vi "Sub_predictor_v3(SubVI).vi"(6 "predicted step":dbl=0.04 format="%#_13g", 8 "Sim_running":bool, 9 "q_i":dbl[](array[numeric]), 11 "t [s]":dbl) -> (0 "Euler Angles Table [deg]":dbl[](array[numeric]), 3 "Euler Angles Table_pred [deg]":dbl[](array[numeric]))   [LabVIEW 2017]
uses:
  <vilib>/Analysis/coordinate.llb/Euler Rotation Order.ctl
  <vilib>/Analysis/7linalg.llb/Real Transpose Matrix.vi
  <vilib>/Analysis/_algsub.llb/Real PseudoInverse Matrix.vi
  <vilib>/Analysis/baseanly.llb/Real A x B.vi
  <vilib>/Analysis/Matrix/Numeric/Conversions/Array To Matrix - RA2.vi
  <vilib>/Analysis/Matrix/Numeric/Conversions/Array To Matrix - RA.vi
  <vilib>/Analysis/Matrix/Numeric/Conversions/Matrix To Array - RM.vi
  <vilib>/Analysis/Matrix/NI_Matrix.lvlib
  <vilib>/Analysis/NI_AALPro.lvlib
  <vilib>/Analysis/NI_AALBase.lvlib
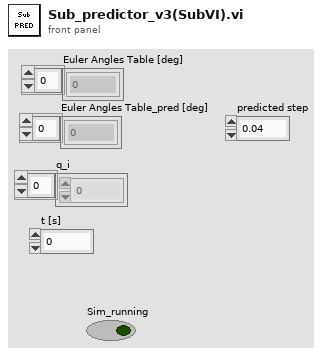
[diagram p1: front panel]
types:
  T1 = typedef "NI_AALPro.lvlib/Euler Rotation Order.ctl" = u16
  T2 = typedef "NI_Matrix.lvlib/RealMatrix.ctl" = dbl[][]
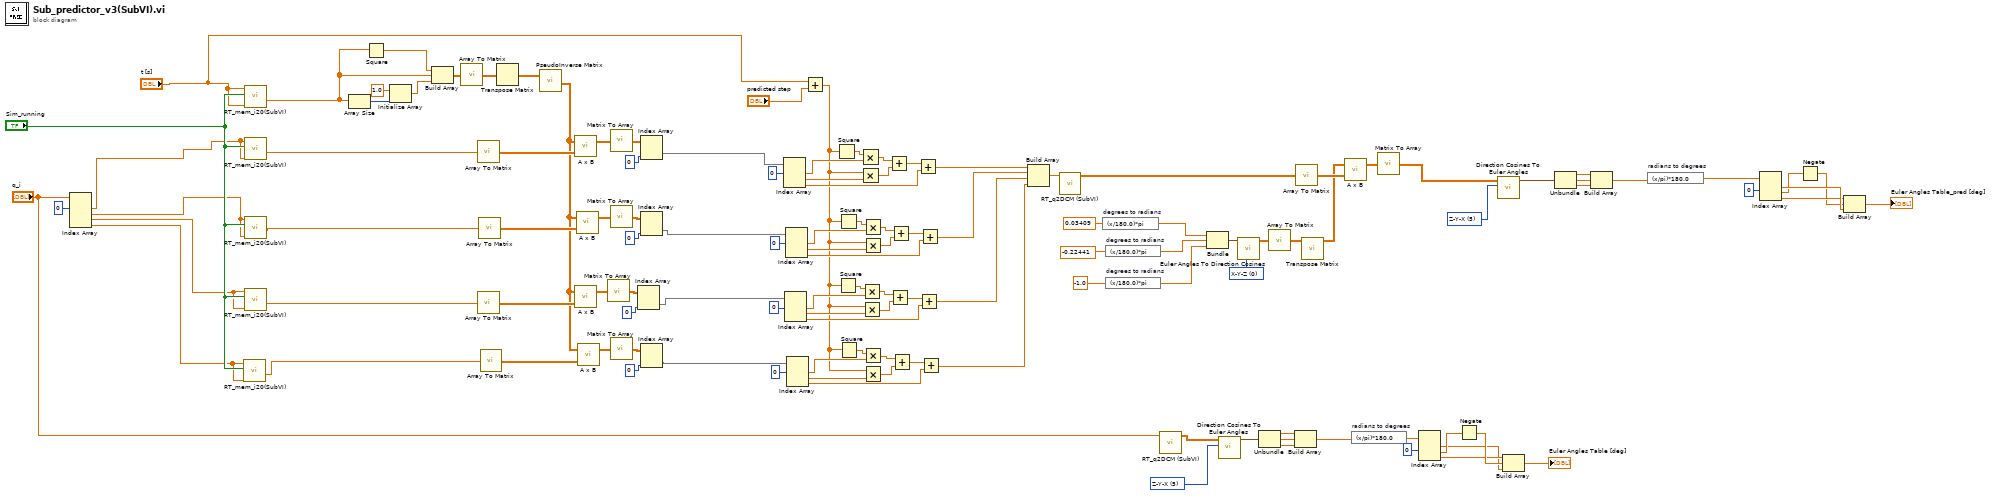
[diagram p0: block diagram]
diagram:
  w14 = T1 0 items=["X-Y-Z", "X-Z-Y", "Y-X-Z", "Y-Z-X", "Z-X-Y", "Z-Y-X", "X-Y-X", "X-Z-X", "Y-X-Y", "Y-Z-Y", "Z-X-Z", "Z-Y-Z"] ("rotation order")
  w17 = T1 5 items=["X-Y-Z", "X-Z-Y", "Y-X-Z", "Y-Z-X", "Z-X-Y", "Z-Y-X", "X-Y-X", "X-Z-X", "Y-X-Y", "Y-Z-Y", "Z-X-Z", "Z-Y-Z"] ("rotation order")
  w43 = T1 5 items=["X-Y-Z", "X-Z-Y", "Y-X-Z", "Y-Z-X", "Z-X-Y", "Z-Y-X", "X-Y-X", "X-Z-X", "Y-X-Y", "Y-Z-Y", "Z-X-Z", "Z-Y-Z"] ("rotation order")
  n1 = Index Array(array="q_i", index #1=0 ("index")) -> (element #1=w92:dbl, element #2=w91:dbl, element #3=w90:dbl, element #4=w89:dbl)  [unwired: 3 in]
  n2 = call "RT_mem_i20(SubVI).vi"("Ini_val"=w89, "start"="Sim_running", "In"=w89) -> ("in_vec"=w95:dbl[])  [unwired: 7 in, 1 out]
  n3 = call "RT_mem_i20(SubVI).vi"("Ini_val"="t [s]", "start"="Sim_running", "In"="t [s]") -> ("in_vec"=w103:dbl[])  [unwired: 7 in, 1 out]
  n4 = call "RT_mem_i20(SubVI).vi"("Ini_val"=w92, "start"="Sim_running", "In"=w92) -> ("in_vec"=w115:dbl[])  [unwired: 7 in, 1 out]
  n5 = call "RT_mem_i20(SubVI).vi"("Ini_val"=w91, "start"="Sim_running", "In"=w91) -> ("in_vec"=w112:dbl[])  [unwired: 7 in, 1 out]
  n6 = call "RT_mem_i20(SubVI).vi"("Ini_val"=w90, "start"="Sim_running", "In"=w90) -> ("in_vec"=w116:dbl[])  [unwired: 7 in, 1 out]
  n7 = Array Size(array=w103) -> (size(s)=w100:i32)
  n8 = Square(x=w103) -> (x^2=w102:dbl[])
  n9 = Initialize Array(1.0 ("element"), w100) -> (w104:dbl[])
  n10 = Build Array(w102, w103, w104) -> (w106:dbl[][])
  n11 = call-poly <vilib>:"Array To Matrix.vi"("Real 2D Array"=w106) -> ("Real Matrix"=w105:T2)
  n12 = call-poly <vilib>:"Array To Matrix.vi"("Real 1D Array"=w115) -> ("Real Matrix (Column Vector)"=w113:T2)
  n13 = call-poly <vilib>:"Array To Matrix.vi"("Real 1D Array"=w116) -> ("Real Matrix (Column Vector)"=w114:T2)
  n14 = call-poly <vilib>:"Array To Matrix.vi"("Real 1D Array"=w112) -> ("Real Matrix (Column Vector)"=w108:T2)
  n15 = call-poly <vilib>:"Array To Matrix.vi"("Real 1D Array"=w95) -> ("Real Matrix (Column Vector)"=w99:T2)
  n16 = Transpose Matrix(1:w105) -> (0:w107:T2)
  n17 = call-poly <vilib>:"PseudoInverse Matrix.vi"("Input Matrix"=w107) -> ("PseudoInverse Matrix"=w94:T2)  [unwired: 1 in, 1 out]
  n18 = call-poly <vilib>:"A x B.vi"("B"=w113, "A"=w94) -> ("A x B"=w121:T2)  [unwired: 1 out]
  n19 = call-poly <vilib>:"A x B.vi"("B"=w114, "A"=w94) -> ("A x B"=w122:T2)  [unwired: 1 out]
  n20 = call-poly <vilib>:"A x B.vi"("B"=w108, "A"=w94) -> ("A x B"=w111:T2)  [unwired: 1 out]
  n21 = call-poly <vilib>:"A x B.vi"("B"=w99, "A"=w94) -> ("A x B"=w96:T2)  [unwired: 1 out]
  n22 = call-poly <vilib>:"Matrix To Array.vi"("Real Matrix"=w122) -> ("Real 2D Array"=w119:dbl[][])
  n23 = call-poly <vilib>:"Matrix To Array.vi"("Real Matrix"=w121) -> ("Real 2D Array"=w118:dbl[][])
  n24 = call-poly <vilib>:"Matrix To Array.vi"("Real Matrix"=w111) -> ("Real 2D Array"=w109:dbl[][])
  n25 = call-poly <vilib>:"Matrix To Array.vi"("Real Matrix"=w96) -> ("Real 2D Array"=w98:dbl[][])
  n26 = Index Array(array=w119, index (col)=0 ("index (row)")) -> (element=w51:dbl[])  [unwired: 1 in]
  n27 = Index Array(array=w118, index (col)=0 ("index (row)")) -> (element=w78:dbl[])  [unwired: 1 in]
  n28 = Index Array(array=w109, index (col)=0 ("index (row)")) -> (element=w52:dbl[])  [unwired: 1 in]
  n29 = Index Array(array=w98, index (col)=0 ("index (row)")) -> (element=w50:dbl[])  [unwired: 1 in]
  n30 = Index Array(array=w78, index #1=0 ("index")) -> (element #1=w81:dbl, element #2=w83:dbl, element #3=w86:dbl)  [unwired: 2 in]
  n31 = Index Array(array=w51, index #1=0 ("index")) -> (element #1=w63:dbl, element #2=w65:dbl, element #3=w68:dbl)  [unwired: 2 in]
  n32 = Index Array(array=w52, index #1=0 ("index")) -> (element #1=w74:dbl, element #2=w72:dbl, element #3=w69:dbl)  [unwired: 2 in]
  n33 = Index Array(array=w50, index #1=0 ("index")) -> (element #1=w58:dbl, element #2=w56:dbl, element #3=w53:dbl)  [unwired: 2 in]
  n34 = Add(x="t [s]", y="predicted step") -> (x+y=w49:dbl)
  n35 = Square(x=w49) -> (x^2=w80:dbl)
  n36 = Square(x=w49) -> (x^2=w62:dbl)
  n37 = Square(x=w49) -> (x^2=w75:dbl)
  n38 = Square(x=w49) -> (x^2=w59:dbl)
  n39 = Multiply(x=w80, y=w81) -> (x*y=w82:dbl)
  n40 = Multiply(x=w49, y=w83) -> (x*y=w84:dbl)
  n41 = Multiply(x=w62, y=w63) -> (x*y=w64:dbl)
  n42 = Multiply(x=w49, y=w65) -> (x*y=w66:dbl)
  n43 = Multiply(x=w75, y=w74) -> (x*y=w73:dbl)
  n44 = Multiply(x=w49, y=w72) -> (x*y=w71:dbl)
  n45 = Multiply(x=w59, y=w58) -> (x*y=w57:dbl)
  n46 = Multiply(x=w49, y=w56) -> (x*y=w55:dbl)
  n47 = Add(x=w82, y=w84) -> (x+y=w85:dbl)
  n48 = Add(x=w64, y=w66) -> (x+y=w67:dbl)
  n49 = Add(x=w73, y=w71) -> (x+y=w70:dbl)
  n50 = Add(x=w57, y=w55) -> (x+y=w54:dbl)
  n51 = Add(x=w85, y=w86) -> (x+y=w48:dbl)
  n52 = Add(x=w67, y=w68) -> (x+y=w46:dbl)
  n53 = Add(x=w70, y=w69) -> (x+y=w47:dbl)
  n54 = Add(x=w54, y=w53) -> (x+y=w45:dbl)
  n55 = Build Array(w48, w47, w46, w45) -> (w44:dbl[])
  n56 = call "RT_q2DCM (SubVI).vi"("Quaternion"=w44) -> ("DCM"=w3:dbl[][])  [unwired: 10 in]
  n57 = expression code="(x/180.0)*pi" "degrees to radians"(0.03409 ("y")) -> (w13:dbl)
  n58 = expression code="(x/180.0)*pi" "degrees to radians"(-0.22441 ("y")) -> (w12:dbl)
  n59 = expression code="(x/180.0)*pi" "degrees to radians"(-1.0 ("y")) -> (w11:dbl)
  n60 = call "RT_q2DCM (SubVI).vi"("Quaternion"="q_i") -> ("DCM"=w22:dbl[][])  [unwired: 10 in]
  n61 = Bundle("y"=w13, "y"=w12, "y"=w11) -> (w15:cluster{"y":dbl, "y":dbl, "y":dbl})  [unwired: 1 in]
  n62 = call <vilib>:"Direction Cosines To Euler Angles.vi"("rotation order"=w17, "Direction Cosines"=w22) -> ("Euler Angles"=w20:cluster{"phi":dbl, "theta":dbl, "psi":dbl})  [unwired: 8 in, 1 out]
  n63 = call <vilib>:"Euler Angles To Direction Cosines.vi"("rotation order"=w14, "Euler Angles"=w15) -> ("Direction Cosines"=w7:dbl[][])  [unwired: 8 in, 1 out]
  n64 = Unbundle(w20) -> ("phi"=w18:dbl, "theta"=w19:dbl, "psi"=w21:dbl)
  n65 = call-poly <vilib>:"Array To Matrix.vi"("Real 2D Array"=w7) -> ("Real Matrix"=w6:T2)
  n66 = Build Array(w18, w19, w21) -> (w30:dbl[])
  n67 = call-poly <vilib>:"Array To Matrix.vi"("Real 2D Array"=w3) -> ("Real Matrix"=w5:T2)
  n68 = call-poly <vilib>:"Transpose Matrix.vi"("Input Matrix"=w6) -> ("Matrix Transpose"=w4:T2)  [unwired: 9 in, 1 out]
  n69 = call-poly <vilib>:"A x B.vi"("B"=w5, "A"=w4) -> ("A x B"=w2:T2)  [unwired: 1 out]
  n70 = expression code="(x/pi)*180.0" "radians to degrees"(w30) -> (w26:dbl[])
  n71 = call-poly <vilib>:"Matrix To Array.vi"("Real Matrix"=w2) -> ("Real 2D Array"=w1:dbl[][])
  n72 = Index Array(array=w26, index #1=0 ("index")) -> (element #1=w24:dbl, element #2=w29:dbl, element #3=w27:dbl)  [unwired: 2 in]
  n73 = Negate(x=w29) -> (-x=w28:dbl)
  n74 = call <vilib>:"Direction Cosines To Euler Angles.vi"("rotation order"=w43, "Direction Cosines"=w1) -> ("Euler Angles"=w40:cluster{"phi":dbl, "theta":dbl, "psi":dbl})  [unwired: 8 in, 1 out]
  n75 = Build Array(w27, w28, w24) -> (→"Euler Angles Table [deg]":dbl[])
  n76 = Unbundle(w40) -> ("phi"=w42:dbl, "theta"=w41:dbl, "psi"=w39:dbl)
  n77 = Build Array(w42, w41, w39) -> (w31:dbl[])
  n78 = expression code="(x/pi)*180.0" "radians to degrees"(w31) -> (w35:dbl[])
  n79 = Index Array(array=w35, index #1=0 ("index")) -> (element #1=w37:dbl, element #2=w32:dbl, element #3=w34:dbl)  [unwired: 2 in]
  n80 = Negate(x=w32) -> (-x=w33:dbl)
  n81 = Build Array(w34, w33, w37) -> (→"Euler Angles Table_pred [deg]":dbl[])
